vi "S4GUI_002.vi"(7 "Tab ObsEng":enum32{"Obs", "CCD modes", "Eng"}(tab)) -> ()   [LabVIEW 2018] (continued)
        n4821 = call-dynamic "Write State Machine.vi"("error in (no error)"=w11600, "State Machine.lvclass"=w11599, "Device in"=w11598) -> ("error out"=w11595:errorcluster, "Device out"=w11597:refnum<class "Opt_Continuous.lvclass">)  [unwired: 7 in]
        n4822 = call "Write GMIR.vi"("error in (no error)"=w11595, "Opt_Continuous.lvclass"=w11597, "Instrument in"=w11596) -> ("error out"=w11592:errorcluster, "Instrument out"=w11594:refnum<class "Instrument.lvclass">)  [unwired: 7 in]
        n4823 = call "Write Instrument.lvclass.vi"("error in (no error)"=w11592, "Instrument.lvclass"=w11594, "S4ACS_GUI in"=w11593) -> ("error out"=w11591:errorcluster, "S4ACS_GUI out"=w11590:refnum<class "S4GUI.lvclass">)  [unwired: 7 in]
      }
      event "GFOC_target": Value Change {
        n4824 = event-data() -> ("NewVal"=w11619:dbl)  [unwired: 1 in, 3 out]
        n4825 = call "Read Instrument.lvclass.vi"("error in (no error)"=w11623, "S4ACS_GUI in"=w11624) -> ("error out"=w11621:errorcluster, "Instrument.lvclass"=w11622:refnum<class "Instrument.lvclass">, "S4ACS_GUI out"=w11613:refnum<class "S4GUI.lvclass">)  [unwired: 7 in]
        n4826 = call "Read GFOC.vi"("error in (no error)"=w11621, "Instrument in"=w11622) -> ("error out"=w11618:errorcluster, "Opt_Continuous.lvclass"=w11620:refnum<class "Opt_Continuous.lvclass">, "Instrument out"=w11616:refnum<class "Instrument.lvclass">)  [unwired: 7 in]
        n4827 = call "Write target.vi"("error in (no error)"=w11618, "target"=w11619, "Optics in"=w11620) -> ("error out"=w11615:errorcluster, "Optics out"=w11617:refnum<class "Opt_Continuous.lvclass">)  [unwired: 7 in]
        n4828 = call "Write GFOC.vi"("error in (no error)"=w11615, "Opt_Continuous.lvclass"=w11617, "Instrument in"=w11616) -> ("error out"=w11612:errorcluster, "Instrument out"=w11614:refnum<class "Instrument.lvclass">)  [unwired: 7 in]
        n4829 = call "Write Instrument.lvclass.vi"("error in (no error)"=w11612, "Instrument.lvclass"=w11614, "S4ACS_GUI in"=w11613) -> ("error out"=w11611:errorcluster, "S4ACS_GUI out"=w11610:refnum<class "S4GUI.lvclass">)  [unwired: 7 in]
      }
      event "GFOC_set": Value Change {
        n4830 = event-data() -> ()  [unwired: 1 in, 4 out]
        n4831 = call "Read Instrument.lvclass.vi"("error in (no error)"=w11643, "S4ACS_GUI in"=w11644) -> ("error out"=w11641:errorcluster, "Instrument.lvclass"=w11642:refnum<class "Instrument.lvclass">, "S4ACS_GUI out"=w11629:refnum<class "S4GUI.lvclass">)  [unwired: 7 in]
        n4832 = call "Read GFOC.vi"("error in (no error)"=w11641, "Instrument in"=w11642) -> ("error out"=w11638:errorcluster, "Opt_Continuous.lvclass"=w11640:refnum<class "Opt_Continuous.lvclass">, "Instrument out"=w11632:refnum<class "Instrument.lvclass">)  [unwired: 7 in]
        n4833 = call-dynamic "Read State Machine.vi"("error in (no error)"=w11638, "Device in"=w11640) -> ("error out"=w11637:errorcluster, "State Machine.lvclass"=w11626:refnum<class "State Machine.lvclass">, "Device out"=w11634:refnum<class "Opt_Continuous.lvclass">)  [unwired: 7 in]
        n4834 = call "Next State.vi"("error in (no error)"=w11637, "New_State"=1, "State Machine in"=w11626) -> ("error out"=w11636:errorcluster, "State Machine out"=w11635:refnum<class "State Machine.lvclass">)  [unwired: 7 in]
        n4835 = call-dynamic "Write State Machine.vi"("error in (no error)"=w11636, "State Machine.lvclass"=w11635, "Device in"=w11634) -> ("error out"=w11631:errorcluster, "Device out"=w11633:refnum<class "Opt_Continuous.lvclass">)  [unwired: 7 in]
        n4836 = call "Write GFOC.vi"("error in (no error)"=w11631, "Opt_Continuous.lvclass"=w11633, "Instrument in"=w11632) -> ("error out"=w11628:errorcluster, "Instrument out"=w11630:refnum<class "Instrument.lvclass">)  [unwired: 7 in]
        n4837 = call "Write Instrument.lvclass.vi"("error in (no error)"=w11628, "Instrument.lvclass"=w11630, "S4ACS_GUI in"=w11629) -> ("error out"=w11627:errorcluster, "S4ACS_GUI out"=w11625:refnum<class "S4GUI.lvclass">)  [unwired: 7 in]
      }
      event "GFOC_stop": Value Change {
        n4838 = event-data() -> ()  [unwired: 1 in, 4 out]
        n4839 = call "Read Instrument.lvclass.vi"("error in (no error)"=w11663, "S4ACS_GUI in"=w11664) -> ("error out"=w11661:errorcluster, "Instrument.lvclass"=w11662:refnum<class "Instrument.lvclass">, "S4ACS_GUI out"=w11648:refnum<class "S4GUI.lvclass">)  [unwired: 7 in]
        n4840 = call "Read GFOC.vi"("error in (no error)"=w11661, "Instrument in"=w11662) -> ("error out"=w11657:errorcluster, "Opt_Continuous.lvclass"=w11660:refnum<class "Opt_Continuous.lvclass">, "Instrument out"=w11651:refnum<class "Instrument.lvclass">)  [unwired: 7 in]
        n4841 = call-dynamic "Read State Machine.vi"("error in (no error)"=w11657, "Device in"=w11660) -> ("error out"=w11656:errorcluster, "State Machine.lvclass"=w11659:refnum<class "State Machine.lvclass">, "Device out"=w11653:refnum<class "Opt_Continuous.lvclass">)  [unwired: 7 in]
        n4842 = call "Next State.vi"("error in (no error)"=w11656, "New_State"=10, "State Machine in"=w11659) -> ("error out"=w11655:errorcluster, "State Machine out"=w11654:refnum<class "State Machine.lvclass">)  [unwired: 7 in]
        n4843 = call-dynamic "Write State Machine.vi"("error in (no error)"=w11655, "State Machine.lvclass"=w11654, "Device in"=w11653) -> ("error out"=w11650:errorcluster, "Device out"=w11652:refnum<class "Opt_Continuous.lvclass">)  [unwired: 7 in]
        n4844 = call "Write GFOC.vi"("error in (no error)"=w11650, "Opt_Continuous.lvclass"=w11652, "Instrument in"=w11651) -> ("error out"=w11647:errorcluster, "Instrument out"=w11649:refnum<class "Instrument.lvclass">)  [unwired: 7 in]
        n4845 = call "Write Instrument.lvclass.vi"("error in (no error)"=w11647, "Instrument.lvclass"=w11649, "S4ACS_GUI in"=w11648) -> ("error out"=w11646:errorcluster, "S4ACS_GUI out"=w11645:refnum<class "S4GUI.lvclass">)  [unwired: 7 in]
      }
      event "GFOC_init": Value Change {
        n4846 = event-data() -> ()  [unwired: 1 in, 4 out]
        n4847 = call "Read Instrument.lvclass.vi"("error in (no error)"=w11683, "S4ACS_GUI in"=w11684) -> ("error out"=w11681:errorcluster, "Instrument.lvclass"=w11682:refnum<class "Instrument.lvclass">, "S4ACS_GUI out"=w11668:refnum<class "S4GUI.lvclass">)  [unwired: 7 in]
        n4848 = call "Read GFOC.vi"("error in (no error)"=w11681, "Instrument in"=w11682) -> ("error out"=w11677:errorcluster, "Opt_Continuous.lvclass"=w11680:refnum<class "Opt_Continuous.lvclass">, "Instrument out"=w11671:refnum<class "Instrument.lvclass">)  [unwired: 7 in]
        n4849 = call-dynamic "Read State Machine.vi"("error in (no error)"=w11677, "Device in"=w11680) -> ("error out"=w11676:errorcluster, "State Machine.lvclass"=w11679:refnum<class "State Machine.lvclass">, "Device out"=w11673:refnum<class "Opt_Continuous.lvclass">)  [unwired: 7 in]
        n4850 = call "Next State.vi"("error in (no error)"=w11676, "New_State"=30, "State Machine in"=w11679) -> ("error out"=w11675:errorcluster, "State Machine out"=w11674:refnum<class "State Machine.lvclass">)  [unwired: 7 in]
        n4851 = call-dynamic "Write State Machine.vi"("error in (no error)"=w11675, "State Machine.lvclass"=w11674, "Device in"=w11673) -> ("error out"=w11670:errorcluster, "Device out"=w11672:refnum<class "Opt_Continuous.lvclass">)  [unwired: 7 in]
        n4852 = call "Write GFOC.vi"("error in (no error)"=w11670, "Opt_Continuous.lvclass"=w11672, "Instrument in"=w11671) -> ("error out"=w11667:errorcluster, "Instrument out"=w11669:refnum<class "Instrument.lvclass">)  [unwired: 7 in]
        n4853 = call "Write Instrument.lvclass.vi"("error in (no error)"=w11667, "Instrument.lvclass"=w11669, "S4ACS_GUI in"=w11668) -> ("error out"=w11666:errorcluster, "S4ACS_GUI out"=w11665:refnum<class "S4GUI.lvclass">)  [unwired: 7 in]
      }
      event "CALW_target": Value Change {
        n4854 = event-data() -> ("NewVal"=w11694:dbl)  [unwired: 1 in, 3 out]
        n4855 = call "Read Instrument.lvclass.vi"("error in (no error)"=w11698, "S4ACS_GUI in"=w11699) -> ("error out"=w11696:errorcluster, "Instrument.lvclass"=w11697:refnum<class "Instrument.lvclass">, "S4ACS_GUI out"=w11688:refnum<class "S4GUI.lvclass">)  [unwired: 7 in]
        n4856 = call "Read CALW.vi"("error in (no error)"=w11696, "Instrument in"=w11697) -> ("error out"=w11693:errorcluster, "Opt_Selector.lvclass"=w11695:refnum<class "Opt_Selector.lvclass">, "Instrument out"=w11691:refnum<class "Instrument.lvclass">)  [unwired: 7 in]
        n4857 = call "Write target.vi"("error in (no error)"=w11693, "target"=w11694, "Optics in"=w11695) -> ("error out"=w11690:errorcluster, "Optics out"=w11692:refnum<class "Opt_Selector.lvclass">)  [unwired: 7 in]
        n4858 = call "Write CALW.vi"("error in (no error)"=w11690, "Opt_Selector.lvclass"=w11692, "Instrument in"=w11691) -> ("error out"=w11687:errorcluster, "Instrument out"=w11689:refnum<class "Instrument.lvclass">)  [unwired: 7 in]
        n4859 = call "Write Instrument.lvclass.vi"("error in (no error)"=w11687, "Instrument.lvclass"=w11689, "S4ACS_GUI in"=w11688) -> ("error out"=w11686:errorcluster, "S4ACS_GUI out"=w11685:refnum<class "S4GUI.lvclass">)  [unwired: 7 in]
      }
      event "CALW_set": Value Change {
        n4860 = event-data() -> ()  [unwired: 1 in, 4 out]
        n4861 = call "Read Instrument.lvclass.vi"("error in (no error)"=w11718, "S4ACS_GUI in"=w11719) -> ("error out"=w11716:errorcluster, "Instrument.lvclass"=w11717:refnum<class "Instrument.lvclass">, "S4ACS_GUI out"=w11704:refnum<class "S4GUI.lvclass">)  [unwired: 7 in]
        n4862 = call "Read CALW.vi"("error in (no error)"=w11716, "Instrument in"=w11717) -> ("error out"=w11713:errorcluster, "Opt_Selector.lvclass"=w11715:refnum<class "Opt_Selector.lvclass">, "Instrument out"=w11707:refnum<class "Instrument.lvclass">)  [unwired: 7 in]
        n4863 = call-dynamic "Read State Machine.vi"("error in (no error)"=w11713, "Device in"=w11715) -> ("error out"=w11712:errorcluster, "State Machine.lvclass"=w11701:refnum<class "State Machine.lvclass">, "Device out"=w11709:refnum<class "Opt_Selector.lvclass">)  [unwired: 7 in]
        n4864 = call "Next State.vi"("error in (no error)"=w11712, "New_State"=1, "State Machine in"=w11701) -> ("error out"=w11711:errorcluster, "State Machine out"=w11710:refnum<class "State Machine.lvclass">)  [unwired: 7 in]
        n4865 = call-dynamic "Write State Machine.vi"("error in (no error)"=w11711, "State Machine.lvclass"=w11710, "Device in"=w11709) -> ("error out"=w11706:errorcluster, "Device out"=w11708:refnum<class "Opt_Selector.lvclass">)  [unwired: 7 in]
        n4866 = call "Write CALW.vi"("error in (no error)"=w11706, "Opt_Selector.lvclass"=w11708, "Instrument in"=w11707) -> ("error out"=w11703:errorcluster, "Instrument out"=w11705:refnum<class "Instrument.lvclass">)  [unwired: 7 in]
        n4867 = call "Write Instrument.lvclass.vi"("error in (no error)"=w11703, "Instrument.lvclass"=w11705, "S4ACS_GUI in"=w11704) -> ("error out"=w11702:errorcluster, "S4ACS_GUI out"=w11700:refnum<class "S4GUI.lvclass">)  [unwired: 7 in]
      }
      event "CALW_stop": Value Change {
        n4868 = event-data() -> ()  [unwired: 1 in, 4 out]
        n4869 = call "Read Instrument.lvclass.vi"("error in (no error)"=w11738, "S4ACS_GUI in"=w11739) -> ("error out"=w11736:errorcluster, "Instrument.lvclass"=w11737:refnum<class "Instrument.lvclass">, "S4ACS_GUI out"=w11723:refnum<class "S4GUI.lvclass">)  [unwired: 7 in]
        n4870 = call "Read CALW.vi"("error in (no error)"=w11736, "Instrument in"=w11737) -> ("error out"=w11732:errorcluster, "Opt_Selector.lvclass"=w11735:refnum<class "Opt_Selector.lvclass">, "Instrument out"=w11726:refnum<class "Instrument.lvclass">)  [unwired: 7 in]
        n4871 = call-dynamic "Read State Machine.vi"("error in (no error)"=w11732, "Device in"=w11735) -> ("error out"=w11731:errorcluster, "State Machine.lvclass"=w11734:refnum<class "State Machine.lvclass">, "Device out"=w11728:refnum<class "Opt_Selector.lvclass">)  [unwired: 7 in]
        n4872 = call "Next State.vi"("error in (no error)"=w11731, "New_State"=10, "State Machine in"=w11734) -> ("error out"=w11730:errorcluster, "State Machine out"=w11729:refnum<class "State Machine.lvclass">)  [unwired: 7 in]
        n4873 = call-dynamic "Write State Machine.vi"("error in (no error)"=w11730, "State Machine.lvclass"=w11729, "Device in"=w11728) -> ("error out"=w11725:errorcluster, "Device out"=w11727:refnum<class "Opt_Selector.lvclass">)  [unwired: 7 in]
        n4874 = call "Write CALW.vi"("error in (no error)"=w11725, "Opt_Selector.lvclass"=w11727, "Instrument in"=w11726) -> ("error out"=w11722:errorcluster, "Instrument out"=w11724:refnum<class "Instrument.lvclass">)  [unwired: 7 in]
        n4875 = call "Write Instrument.lvclass.vi"("error in (no error)"=w11722, "Instrument.lvclass"=w11724, "S4ACS_GUI in"=w11723) -> ("error out"=w11721:errorcluster, "S4ACS_GUI out"=w11720:refnum<class "S4GUI.lvclass">)  [unwired: 7 in]
      }
      event "CALW_init": Value Change {
        n4876 = event-data() -> ()  [unwired: 1 in, 4 out]
        n4877 = call "Read Instrument.lvclass.vi"("error in (no error)"=w11758, "S4ACS_GUI in"=w11759) -> ("error out"=w11756:errorcluster, "Instrument.lvclass"=w11757:refnum<class "Instrument.lvclass">, "S4ACS_GUI out"=w11743:refnum<class "S4GUI.lvclass">)  [unwired: 7 in]
        n4878 = call "Read CALW.vi"("error in (no error)"=w11756, "Instrument in"=w11757) -> ("error out"=w11752:errorcluster, "Opt_Selector.lvclass"=w11755:refnum<class "Opt_Selector.lvclass">, "Instrument out"=w11746:refnum<class "Instrument.lvclass">)  [unwired: 7 in]
        n4879 = call-dynamic "Read State Machine.vi"("error in (no error)"=w11752, "Device in"=w11755) -> ("error out"=w11751:errorcluster, "State Machine.lvclass"=w11754:refnum<class "State Machine.lvclass">, "Device out"=w11748:refnum<class "Opt_Selector.lvclass">)  [unwired: 7 in]
        n4880 = call "Next State.vi"("error in (no error)"=w11751, "New_State"=30, "State Machine in"=w11754) -> ("error out"=w11750:errorcluster, "State Machine out"=w11749:refnum<class "State Machine.lvclass">)  [unwired: 7 in]
        n4881 = call-dynamic "Write State Machine.vi"("error in (no error)"=w11750, "State Machine.lvclass"=w11749, "Device in"=w11748) -> ("error out"=w11745:errorcluster, "Device out"=w11747:refnum<class "Opt_Selector.lvclass">)  [unwired: 7 in]
        n4882 = call "Write CALW.vi"("error in (no error)"=w11745, "Opt_Selector.lvclass"=w11747, "Instrument in"=w11746) -> ("error out"=w11742:errorcluster, "Instrument out"=w11744:refnum<class "Instrument.lvclass">)  [unwired: 7 in]
        n4883 = call "Write Instrument.lvclass.vi"("error in (no error)"=w11742, "Instrument.lvclass"=w11744, "S4ACS_GUI in"=w11743) -> ("error out"=w11741:errorcluster, "S4ACS_GUI out"=w11740:refnum<class "S4GUI.lvclass">)  [unwired: 7 in]
      }
      event "ASEL_target": Value Change {
        n4884 = event-data() -> ("NewVal"=w11769:dbl)  [unwired: 1 in, 3 out]
        n4885 = call "Read Instrument.lvclass.vi"("error in (no error)"=w11773, "S4ACS_GUI in"=w11774) -> ("error out"=w11771:errorcluster, "Instrument.lvclass"=w11772:refnum<class "Instrument.lvclass">, "S4ACS_GUI out"=w11763:refnum<class "S4GUI.lvclass">)  [unwired: 7 in]
        n4886 = call "Read ASEL.vi"("error in (no error)"=w11771, "Instrument in"=w11772) -> ("error out"=w11768:errorcluster, "Opt_Selector.lvclass"=w11770:refnum<class "Opt_Selector.lvclass">, "Instrument out"=w11766:refnum<class "Instrument.lvclass">)  [unwired: 7 in]
        n4887 = call "Write target.vi"("error in (no error)"=w11768, "target"=w11769, "Optics in"=w11770) -> ("error out"=w11765:errorcluster, "Optics out"=w11767:refnum<class "Opt_Selector.lvclass">)  [unwired: 7 in]
        n4888 = call "Write ASEL.vi"("error in (no error)"=w11765, "Opt_Selector.lvclass"=w11767, "Instrument in"=w11766) -> ("error out"=w11762:errorcluster, "Instrument out"=w11764:refnum<class "Instrument.lvclass">)  [unwired: 7 in]
        n4889 = call "Write Instrument.lvclass.vi"("error in (no error)"=w11762, "Instrument.lvclass"=w11764, "S4ACS_GUI in"=w11763) -> ("error out"=w11761:errorcluster, "S4ACS_GUI out"=w11760:refnum<class "S4GUI.lvclass">)  [unwired: 7 in]
      }
      event "ASEL_set": Value Change {
        n4890 = event-data() -> ()  [unwired: 1 in, 4 out]
        n4891 = call "Read Instrument.lvclass.vi"("error in (no error)"=w11793, "S4ACS_GUI in"=w11794) -> ("error out"=w11791:errorcluster, "Instrument.lvclass"=w11792:refnum<class "Instrument.lvclass">, "S4ACS_GUI out"=w11779:refnum<class "S4GUI.lvclass">)  [unwired: 7 in]
        n4892 = call "Read ASEL.vi"("error in (no error)"=w11791, "Instrument in"=w11792) -> ("error out"=w11788:errorcluster, "Opt_Selector.lvclass"=w11790:refnum<class "Opt_Selector.lvclass">, "Instrument out"=w11782:refnum<class "Instrument.lvclass">)  [unwired: 7 in]
        n4893 = call-dynamic "Read State Machine.vi"("error in (no error)"=w11788, "Device in"=w11790) -> ("error out"=w11787:errorcluster, "State Machine.lvclass"=w11776:refnum<class "State Machine.lvclass">, "Device out"=w11784:refnum<class "Opt_Selector.lvclass">)  [unwired: 7 in]
        n4894 = call "Next State.vi"("error in (no error)"=w11787, "New_State"=1, "State Machine in"=w11776) -> ("error out"=w11786:errorcluster, "State Machine out"=w11785:refnum<class "State Machine.lvclass">)  [unwired: 7 in]
        n4895 = call-dynamic "Write State Machine.vi"("error in (no error)"=w11786, "State Machine.lvclass"=w11785, "Device in"=w11784) -> ("error out"=w11781:errorcluster, "Device out"=w11783:refnum<class "Opt_Selector.lvclass">)  [unwired: 7 in]
        n4896 = call "Write ASEL.vi"("error in (no error)"=w11781, "Opt_Selector.lvclass"=w11783, "Instrument in"=w11782) -> ("error out"=w11778:errorcluster, "Instrument out"=w11780:refnum<class "Instrument.lvclass">)  [unwired: 7 in]
        n4897 = call "Write Instrument.lvclass.vi"("error in (no error)"=w11778, "Instrument.lvclass"=w11780, "S4ACS_GUI in"=w11779) -> ("error out"=w11777:errorcluster, "S4ACS_GUI out"=w11775:refnum<class "S4GUI.lvclass">)  [unwired: 7 in]
      }
      event "ASEL_stop": Value Change {
        n4898 = event-data() -> ()  [unwired: 1 in, 4 out]
        n4899 = call "Read Instrument.lvclass.vi"("error in (no error)"=w11813, "S4ACS_GUI in"=w11814) -> ("error out"=w11811:errorcluster, "Instrument.lvclass"=w11812:refnum<class "Instrument.lvclass">, "S4ACS_GUI out"=w11798:refnum<class "S4GUI.lvclass">)  [unwired: 7 in]
        n4900 = call "Read ASEL.vi"("error in (no error)"=w11811, "Instrument in"=w11812) -> ("error out"=w11807:errorcluster, "Opt_Selector.lvclass"=w11810:refnum<class "Opt_Selector.lvclass">, "Instrument out"=w11801:refnum<class "Instrument.lvclass">)  [unwired: 7 in]
        n4901 = call-dynamic "Read State Machine.vi"("error in (no error)"=w11807, "Device in"=w11810) -> ("error out"=w11806:errorcluster, "State Machine.lvclass"=w11809:refnum<class "State Machine.lvclass">, "Device out"=w11803:refnum<class "Opt_Selector.lvclass">)  [unwired: 7 in]
        n4902 = call "Next State.vi"("error in (no error)"=w11806, "New_State"=10, "State Machine in"=w11809) -> ("error out"=w11805:errorcluster, "State Machine out"=w11804:refnum<class "State Machine.lvclass">)  [unwired: 7 in]
        n4903 = call-dynamic "Write State Machine.vi"("error in (no error)"=w11805, "State Machine.lvclass"=w11804, "Device in"=w11803) -> ("error out"=w11800:errorcluster, "Device out"=w11802:refnum<class "Opt_Selector.lvclass">)  [unwired: 7 in]
        n4904 = call "Write ASEL.vi"("error in (no error)"=w11800, "Opt_Selector.lvclass"=w11802, "Instrument in"=w11801) -> ("error out"=w11797:errorcluster, "Instrument out"=w11799:refnum<class "Instrument.lvclass">)  [unwired: 7 in]
        n4905 = call "Write Instrument.lvclass.vi"("error in (no error)"=w11797, "Instrument.lvclass"=w11799, "S4ACS_GUI in"=w11798) -> ("error out"=w11796:errorcluster, "S4ACS_GUI out"=w11795:refnum<class "S4GUI.lvclass">)  [unwired: 7 in]
      }
      event "ASEL_init": Value Change {
        n4906 = event-data() -> ()  [unwired: 1 in, 4 out]
        n4907 = call "Read Instrument.lvclass.vi"("error in (no error)"=w11833, "S4ACS_GUI in"=w11834) -> ("error out"=w11831:errorcluster, "Instrument.lvclass"=w11832:refnum<class "Instrument.lvclass">, "S4ACS_GUI out"=w11818:refnum<class "S4GUI.lvclass">)  [unwired: 7 in]
        n4908 = call "Read ASEL.vi"("error in (no error)"=w11831, "Instrument in"=w11832) -> ("error out"=w11827:errorcluster, "Opt_Selector.lvclass"=w11830:refnum<class "Opt_Selector.lvclass">, "Instrument out"=w11821:refnum<class "Instrument.lvclass">)  [unwired: 7 in]
        n4909 = call-dynamic "Read State Machine.vi"("error in (no error)"=w11827, "Device in"=w11830) -> ("error out"=w11826:errorcluster, "State Machine.lvclass"=w11829:refnum<class "State Machine.lvclass">, "Device out"=w11823:refnum<class "Opt_Selector.lvclass">)  [unwired: 7 in]
        n4910 = call "Next State.vi"("error in (no error)"=w11826, "New_State"=30, "State Machine in"=w11829) -> ("error out"=w11825:errorcluster, "State Machine out"=w11824:refnum<class "State Machine.lvclass">)  [unwired: 7 in]
        n4911 = call-dynamic "Write State Machine.vi"("error in (no error)"=w11825, "State Machine.lvclass"=w11824, "Device in"=w11823) -> ("error out"=w11820:errorcluster, "Device out"=w11822:refnum<class "Opt_Selector.lvclass">)  [unwired: 7 in]
        n4912 = call "Write ASEL.vi"("error in (no error)"=w11820, "Opt_Selector.lvclass"=w11822, "Instrument in"=w11821) -> ("error out"=w11817:errorcluster, "Instrument out"=w11819:refnum<class "Instrument.lvclass">)  [unwired: 7 in]
        n4913 = call "Write Instrument.lvclass.vi"("error in (no error)"=w11817, "Instrument.lvclass"=w11819, "S4ACS_GUI in"=w11818) -> ("error out"=w11816:errorcluster, "S4ACS_GUI out"=w11815:refnum<class "S4GUI.lvclass">)  [unwired: 7 in]
      }
    }
    n4914 = Unbundle By Name(w116) -> ("status"=w115:bool)
    n4915 = flat-sequence {
      tunnel: w130 -> [w145]
      tunnel: w128 -> [w143]
      tunnel: [w145] -> w127
      tunnel: [w141] -> w126
      tunnel: [w140] -> w125
      tunnel: [w148] -> w129
      tunnel: w127 -> [w148]
      tunnel: w126 -> [w147]
      tunnel: w125 -> [w146]
      frame #0 {
        n4916 = Tick Count (ms)() -> (millisecond timer value=w144:u32)
        n4917 = local read "loop max(ms)"() -> (w139:u32)
        n4918 = Subtract(x=w144, y=w143) -> (x-y=w141:u32)
        n4919 = Greater?(x=w141, y=w139) -> (0:w142:bool)
        n4920 = Select(t=w141, s=w142, f=w139) -> (s? t:f=w140:u32)
      }
      frame #1 {
        "loop time(ms)" <- w147
        "loop max(ms)" <- w146
      }
    }
    n4921 = Or(x=w115, y=w114) -> (x .or. y?=w113:bool)
  }
  "error out 9" <- w2
  n4922 = while {
    tunnel: w9 -> [_]
    stop <- FALSE stop-if-true
    n4923 = call "ZeroMQ_ACS1.vi"() -> ()  [unwired: 12 in]
    n4924 = call "ZeroMQ_ACS2.vi"() -> ()  [unwired: 12 in]
    n4925 = call "ZeroMQ_ACS3.vi"() -> ()  [unwired: 12 in]
    n4926 = call "ZeroMQ_ACS4.vi"() -> ()  [unwired: 12 in]
    n4927 = disable-structure shown="Enabled" {
      frame Disabled {
        n4928 = call "ZeroMQ_FOC.vi"() -> ()  [unwired: 12 in]
      }
      frame Enabled {
        n4929 = call "ZeroMQ_FOC_REQREP.vi"() -> ()  [unwired: 12 in]
      }
    }
    n4930 = call "ZeroMQ_WSTA.vi"() -> ()  [unwired: 12 in]
    n4931 = call "ZeroMQ_TCS.vi"() -> ()  [unwired: 12 in]
    n4932 = call "ZeroMQ_S4ICS.vi"() -> ()  [unwired: 12 in]
    n4933 = call "ZeroMQ_SUBGS.vi"() -> ()  [unwired: 12 in]
    n4934 = call "StreamTransmitSyncBox.vi"() -> ()  [unwired: 12 in]
    n4935 = call "StreamReceiveSyncBox.vi"() -> ()  [unwired: 12 in]
    n4936 = call "ZeroMQ_PUB.vi"() -> ()  [unwired: 12 in]
  }
  n4937 = stacked-sequence "INTERFACE" {
    frame #0 {
    }
    frame #1 {
    }
    frame #2 {
    }
    frame #3 {
    }
    frame #4 {
    }
  }
  n4938 = call-dynamic "Log Error.vi"("error in (no error)"=w2, "S4GUI in"=w4) -> ("error out"=→"error out 10":errorcluster, "S4GUI out"=w3:refnum<class "S4GUI.lvclass">)  [unwired: 8 in]
  n4939 = call-dynamic "End.vi"("S4ACS_GUI in"=w3) -> ("error out"=w21:errorcluster)  [unwired: 9 in, 1 out]
  n4940 = flat-sequence {
    tunnel: [w11837] -> w19
    tunnel: w21 -> [w11839]
    tunnel: [w11845] -> w20
    tunnel: w19 -> [w11845]
    frame #0 {
      w11843 = FALSE
      # "Apaga todos os leds, habilita Tab ObsEng."
      n4941 = property on="Tab ObsEng" class="TabCtl (strict)"("Tabs Visible?"=TRUE) -> ()  [unwired: 2 in, 2 out]
      n4942 = property on="Channel 4" class="Bool (strict)"("Value"=w11843) -> ()  [unwired: 2 in, 2 out]
      n4943 = property on="Channel 3" class="Bool (strict)"("Value"=w11843) -> ()  [unwired: 2 in, 2 out]
      n4944 = property on="Channel 2" class="Bool (strict)"("Value"=w11843) -> ()  [unwired: 2 in, 2 out]
      n4945 = property on="Channel 1" class="Bool (strict)"("Value"=w11843) -> ()  [unwired: 2 in, 2 out]
      n4946 = property on="S4ICSoft" class="Bool (strict)"("Value"=w11843) -> ()  [unwired: 2 in, 2 out]
      n4947 = call <vilib>:"Clear Errors.vi"("error in (no error)"=w11839) -> ("error out"=w11836:errorcluster)  [unwired: 5 in, 1 out]
      n4948 = property on="TCSPD" class="Bool (strict)"("Value"=w11843) -> ()  [unwired: 2 in, 2 out]
      n4949 = property on="Focus 160" class="Bool (strict)"("Value"=w11843) -> ()  [unwired: 2 in, 2 out]
      n4950 = property on="Weather" class="Bool (strict)"("Value"=w11843) -> ()  [unwired: 2 in, 2 out]
      n4951 = property on="GUIDER" class="Bool (strict)"("Value"=w11843) -> ()  [unwired: 2 in, 2 out]
      n4952 = disable-structure shown="Disabled" {
        frame Disabled {
          n4953 = local write "Last Error"("" ("Last Error")) -> ()
        }
        frame Enabled {
        }
      }
      n4954 = property on="Last Error" class="Str"(error in=w11836, "Text.BG Color"=u32 13816530 ("Color Box"), "Caption.FontBold"=FALSE ("Caption.Font:Bold")) -> (error out=w11838:errorcluster)  [unwired: 1 in, 1 out]
      n4955 = call <vilib>:"Clear Errors.vi"("error in (no error)"=w11838) -> ("error out"=w11837:errorcluster)  [unwired: 5 in, 1 out]
    }
    frame #1 {
      n4956 = Stop() -> ()  [unwired: 1 in]
    }
  }
  "error out" <- w20
  "GUI version" <- w22
